vi "JPL Elevator Control.vi"(9 "Button Control":T2, 10 "Limit Switches":T1) -> (1 "Index":dbl, 3 "Elevator Height":dbl)   [LabVIEW 2014]
uses:
  <vilib>/functionblocks/Edge Detection/One Shot Falling With Input/One Shot Falling With Input.vi
  <vilib>/functionblocks/Edge Detection/One Shot Rising with Input/One Shot Rising with Input.vi
  <vilib>/functionblocks/FB Core/FB Core.xnode
  <vilib>/functionblocks/NI_FunctionBlock Libraries.lvlib
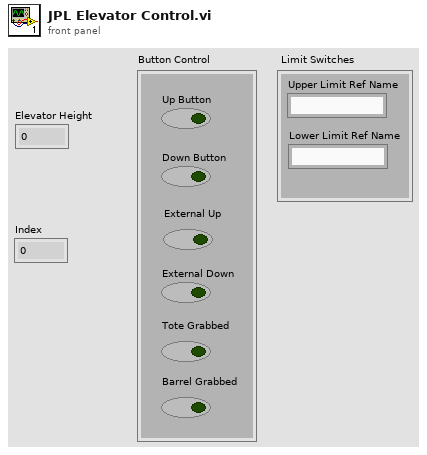
[diagram p1: front panel]
types:
  T1 = cluster{"Upper Limit Ref Name":string, "Lower Limit Ref Name":string}
  T2 = cluster{"Down Button":bool, "Up Button":bool, "External Down":bool, "External Up":bool, "Tote Grabbed":bool, "Barrel Grabbed":bool}
  T3 = typedef "WPI_DigitalInputDevRef.ctl" = cluster{"DevStatus":errorcluster, "DIO Channel":T4, "Controller":T5}
  T4 = typedef "FPGA_DIOChannel.ctl" = enum8{"DIO 0", "DIO 1", "DIO 2", "DIO 3", "DIO 4", "DIO 5", "DIO 6", "DIO 7", "DIO 8", "DIO 9", "DIO MXP 0", "DIO MXP 1", "DIO MXP 2", "DIO MXP 3", "DIO MXP 4", "DIO MXP 5", "DIO MXP 6", "DIO MXP 7", "DIO MXP 8", "DIO MXP 9", "DIO MXP 10", "DIO MXP 11", "DIO MXP 12", "DIO MXP 13", "DIO MXP 14", "DIO MXP 15", "Invalid"}
  T5 = typedef "FPGA_TypedefDigitalModule.ctl" = enum16{"Controller 1"}
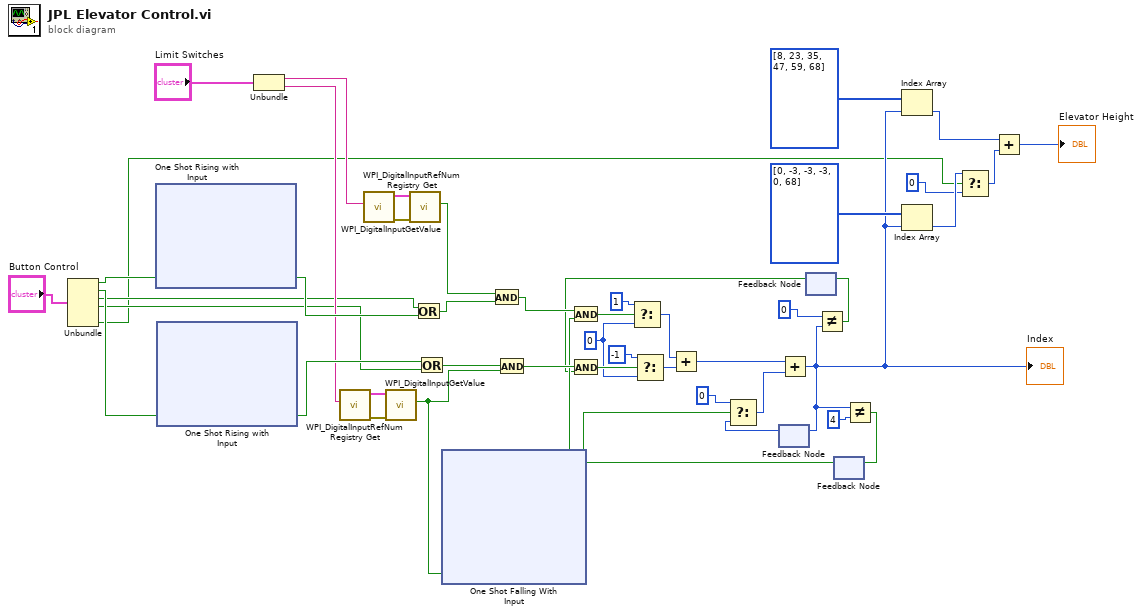
[diagram p0: block diagram]
diagram:
  w27 = 0
  n1 = Unbundle("Button Control") -> ("Down Button"=w20:bool, "Up Button"=w19:bool, "External Down"=w18:bool, "External Up"=w17:bool, "Barrel Grabbed"=w3:bool)  [unwired: 1 out]
  n2 = xnode "One Shot Rising with Input"("input"=w20) -> ("output"=w46:bool)  [unwired: 1 in, 1 out]
  n3 = xnode "One Shot Rising with Input"("input"=w19) -> ("output"=w47:bool)  [unwired: 1 in, 1 out]
  n4 = Unbundle("Limit Switches") -> ("Upper Limit Ref Name"=w23:string, "Lower Limit Ref Name"=w22:string)
  n5 = call <vilib>:"WPI_DigitalInputRefNum Registry Get.vi"("refnum name"=w22) -> ("error out"=w39:errorcluster, "DigitalInputDevRef"=w38:T3)  [unwired: 9 in]
  n6 = call <vilib>:"WPI_DigitalInputRefNum Registry Get.vi"("refnum name"=w23) -> ("error out"=w41:errorcluster, "DigitalInputDevRef"=w40:T3)  [unwired: 9 in]
  n7 = call <vilib>:"WPI_DigitalInputGetValue.vi"("error in (no error)"=w39, "DigitalInputDevRef"=w38) -> ("Value"=w2:bool)  [unwired: 7 in, 2 out]
  n8 = call <vilib>:"WPI_DigitalInputGetValue.vi"("error in (no error)"=w41, "DigitalInputDevRef"=w40) -> ("Value"=w16:bool)  [unwired: 7 in, 2 out]
  n9 = Or(x=w18, y=w46) -> (x .or. y?=w44:bool)
  n10 = Or(x=w47, y=w17) -> (x .or. y?=w42:bool)
  n11 = xnode "One Shot Falling With Input"("input"=w2) -> ("output"=w1:bool)  [unwired: 1 in, 1 out]
  n12 = And(x=w16, y=w44) -> (x .and. y?=w45:bool)
  n13 = And(x=w42, y=w2) -> (x .and. y?=w43:bool)
  n14 = feedback #1() -> (w13:i32)  [unwired: 1 in]
  n15 = Select(t=0, s=w1, f=w13) -> (s? t:f=w14:i32)
  n16 = feedback #2() -> (w34:bool)  [unwired: 1 in]
  n17 = And(x=w43, y=w34) -> (x .and. y?=w31:bool)
  n18 = Select(t=-1, s=w31, f=w27) -> (s? t:f=w25:i32)
  n19 = feedback #3() -> (w36:bool)  [unwired: 1 in]
  n20 = And(x=w45, y=w36) -> (x .and. y?=w30:bool)
  n21 = Select(t=1, s=w30, f=w27) -> (s? t:f=w26:i32)
  n22 = Add(x=w26, y=w25) -> (x+y=w15:i32)
  n23 = Add(x=w15, y=w14) -> (x+y=w9:i32)
  "Index" <- w9
  n24 = feedback-in #1(w9) -> ()
  n25 = Not Equal?(x=0, y=w9) -> (x != y?=w33:bool)
  n26 = feedback-in #2(w33) -> ()
  n27 = Not Equal?(x=w9, y=4) -> (x != y?=w35:bool)
  n28 = feedback-in #3(w35) -> ()
  n29 = Index Array(array=i32[] [8, 23, 35, 47, 59, 68], index=w9) -> (element=w8:i32)
  n30 = Index Array(array=i32[] [0, -3, -3, -3, 0, 68], index=w9) -> (element=w6:i32)
  n31 = Select(t=w6, s=w3, f=0) -> (s? t:f=w7:i32)
  n32 = Add(x=w8, y=w7) -> (x+y=→"Elevator Height":i32)
